vi "Read Position.vi"(0 "reference in":refnum<class "SmartMotor.lvclass">, 5 "error in (no error)":errorcluster) -> (11 "Motor Absolute Position (rev)":dbl, 13 "Motor Relative Position (rev)":dbl, 14 "reference out":refnum<class "SmartMotor.lvclass">, 17 "Motor Absolute Position":i32, 18 "Motor Relative Position (From Last Move)":i32, 19 "error out":errorcluster)   [LabVIEW 2017, in "SmartMotor.lvclass"]
uses:
  SmartMotor.lvclass
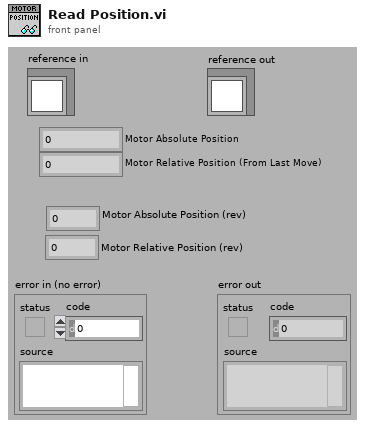
[diagram p1: front panel]
types:
  T1 = typedef "SmartMotor.lvclass/ObjectAttributes.ctl" = cluster{"SmartMotor Chain VISA Resource":refnum<visa-resource-name>, "SmartMotor Chain Address":i16, "Motor Absolute Position":i32, "Motor Relative Position":i32, "Motor Torque":i32, "Motor Voltage":i32, "Screwdriver Engaged":bool, "Screwdriver Torque Limit":i32, "Torque Monitor On/Off Status":bool, "Torque Monitor VI Reference":refnum<vi>, "Absolute Motor Torque (Filtered)":dbl, "SmartMotor Status":T2, "SmartMotor Error":T3}
  T2 = typedef "SmartMotor.lvclass/SmartMotor Status.ctl" = enum8{"Stopped", "Moving"}
  T3 = typedef "SmartMotor.lvclass/SmartMotor Error.ctl" = enum8{"None", "Read Error", "Low Voltage"}
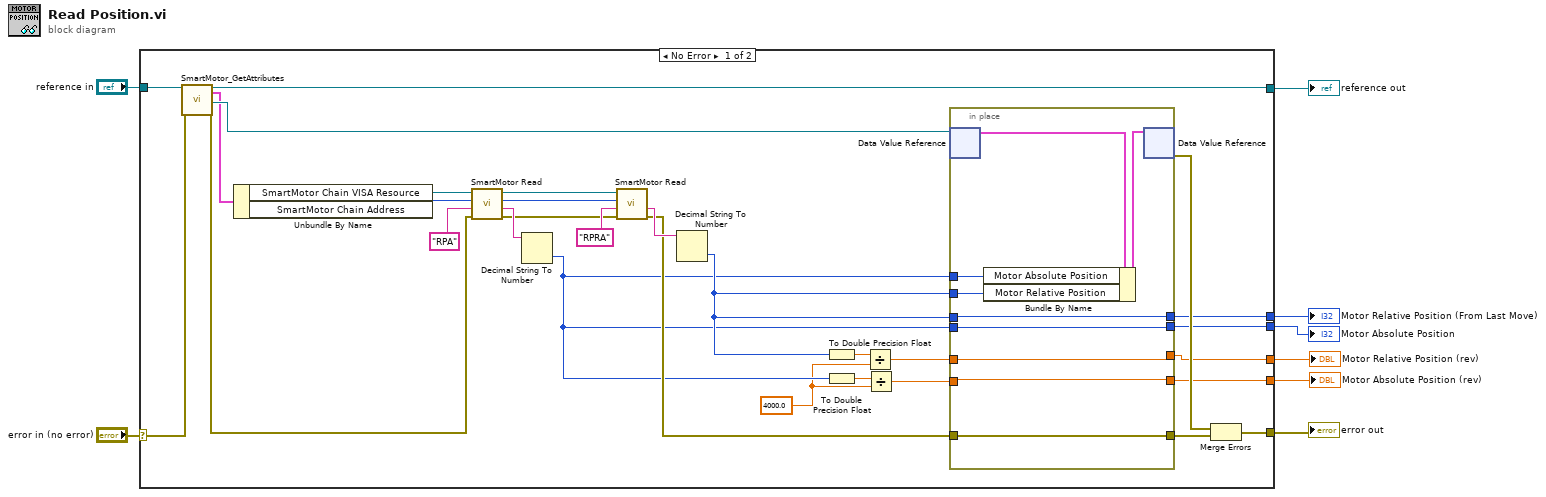
[diagram p0: block diagram]
diagram:
  n1 = case shown="No Error" "error in (no error)" {
    selector: "error in (no error)" -> [w37 w49]
    tunnel: [w35 w49] -> w7
    tunnel: [w36 w48] -> w5
    tunnel: "reference in" -> [w38 w48]
    tunnel: [w31 _] -> w4
    tunnel: [w30 _] -> w3
    tunnel: [w11 _] -> w2
    tunnel: [w9 _] -> w1
    frame No Error {
      w13 = 4000.0
      n2 = call "SmartMotor_GetAttributes.vi"("reference in"=w38, "error in (no error)"=w37) -> ("reference out"=w36:refnum<class "SmartMotor.lvclass">, "Data"=w18:T1, "DataRef"=w34:refnum<data-value>, "error out"=w20:errorcluster)  [unwired: 14 in]
      n3 = Unbundle By Name(w18) -> ("SmartMotor Chain VISA Resource"=w27:refnum<visa-resource-name>, "SmartMotor Chain Address"=w22:i16)
      n4 = call "SmartMotor Read.vi"("VISA resource IN"=w27, "Motor Number"=w22, "Read Command to Motor"="RPA", "Error In"=w20) -> ("VISA resource OUT"=w26:refnum<visa-resource-name>, "Motor Number OUT"=w21:i16, "Response From Motor"=w28:string, "Error Out"=w23:errorcluster)  [unwired: 1 in, 1 out]
      n5 = Decimal String To Number(string=w28) -> (number=w16:i32)  [unwired: 2 in, 1 out]
      n6 = call "SmartMotor Read.vi"("VISA resource IN"=w26, "Motor Number"=w21, "Read Command to Motor"="RPRA", "Error In"=w23) -> ("Response From Motor"=w24:string, "Error Out"=w19:errorcluster)  [unwired: 1 in, 3 out]
      n7 = Decimal String To Number(string=w24) -> (number=w17:i32)  [unwired: 2 in, 1 out]
      n8 = To Double Precision Float(number=w17) -> (double precision float=w15:dbl)
      n9 = To Double Precision Float(number=w16) -> (double precision float=w14:dbl)
      n10 = Divide(x=w15, y=w13) -> (x/y=w12:dbl)
      n11 = Divide(x=w14, y=w13) -> (x/y=w10:dbl)
      n12 = in-place {
        in-place-border: w19 -> [w43]
        in-place-border: [w43] -> w33
        in-place-border: [w41] -> w31
        in-place-border: [w42] -> w30
        in-place-border: w16 -> [w45]
        in-place-border: w17 -> [w44]
        in-place-border: w17 -> [w42]
        in-place-border: w16 -> [w41]
        in-place-border: w12 -> [w40]
        in-place-border: [w40] -> w11
        in-place-border: [w39] -> w9
        in-place-border: w10 -> [w39]
        n13 = in-place-dvr #1(w34) -> (w46:T1)  [unwired: 1 out]
        n14 = Bundle By Name(cluster=w46, "Motor Absolute Position"=w45, "Motor Relative Position"=w44) -> (w47:T1)
        n15 = in-place-dvr #1(w47) -> (w32:errorcluster)  [unwired: 1 out]
      }
      n16 = Merge Errors(w32, w33) -> (w35:errorcluster)
    }
    frame Error {
    }
  }
  "error out" <- w7
  "reference out" <- w5
  "Motor Absolute Position" <- w4
  "Motor Relative Position (From Last Move)" <- w3
  "Motor Relative Position (rev)" <- w2
  "Motor Absolute Position (rev)" <- w1
